vi "Parse VIPM Filename.vi"(9 "Filename":string) -> (4 "edition":string, 5 "version":string)   [LabVIEW 2014, in "Raspberry Pi Compatible Compiler for LabVIEW.lvlib"]
uses:
  <vilib>/regexp/Match Regular Expression.xnode
  Raspberry Pi Compatible Compiler for LabVIEW.lvlib
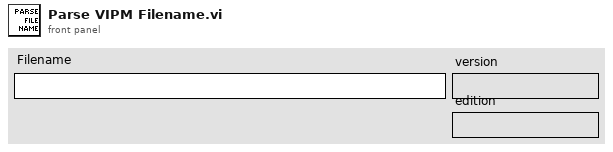
[diagram p1: front panel]
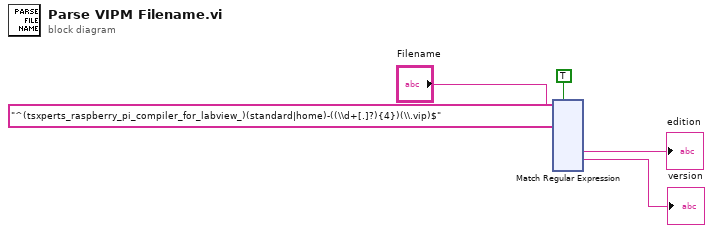
[diagram p0: block diagram]
diagram:
  n1 = xnode "Match Regular Expression"("input string"="Filename", "regular expression"="^(tsxperts_raspberry_pi_compiler_for_labview_)(standard|home)-((\\d+[.]?){4})(\\.vip)$", "ignore case? (F)"=TRUE) -> ("submatch 2"=→"edition":string, "submatch 3"=→"version":string)  [unwired: 3 in, 7 out]
